vi "SetTaskList.vi"(8 "error in (no error)":errorcluster, 10 "OrderedList":refnum<class "Collection.lvclass">, 11 "OrderedList in":refnum<class "TaskList.lvclass">) -> (0 "error out":errorcluster, 3 "OrderedList out":refnum<class "TaskList.lvclass">)   [LabVIEW 2021, in "LvMarkdown.lvlib" / "TaskList.lvclass"]
uses:
  TaskList.lvclass
  Collection/Collection.lvclass
  TaskList.lvclass/TaskList.ctl
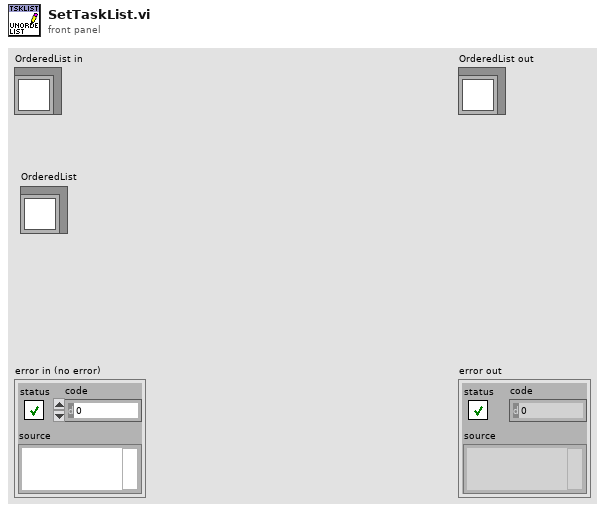
[diagram p1: front panel]
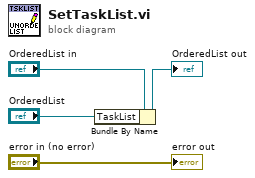
[diagram p0: block diagram]
diagram:
  n1 = Bundle By Name(cluster="OrderedList in", "TaskList"="OrderedList") -> (→"OrderedList out":refnum<class "TaskList.lvclass">)
  "error out" <- "error in (no error)"
